vi "GT Get Dac Config.vi"(8 "error in (no error)":errorcluster caption="错误输入（无错误）", 9 "pDac":T1, 10 "dac":i16, 11 "cardNum":i16) -> (0 "error out":errorcluster caption="错误输出", 1 "pDac out":T1, 3 "function return":i16)   [LabVIEW 2020, in "gts1.lvlib"]
doc: "GT_API GT_GetDacConfig(short cardNum,short dac,TDacConfig *pDac);"
uses:
  gts1.lvlib
  dll/32bit/multi_card/gts.dll
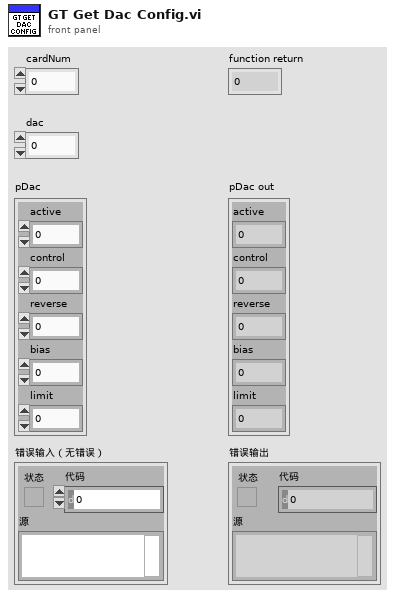
[diagram p1: front panel]
types:
  T1 = cluster{"active":i16, "control":i16, "reverse":i16, "bias":i16, "limit":i16}
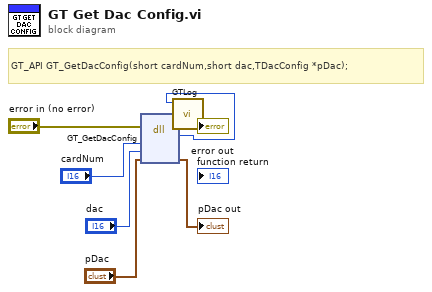
[diagram p0: block diagram]
diagram:
  # "GT_API GT_GetDacConfig(short cardNum,short dac,TDacConfig *pDac);"
  n1 = dll-call lib="C:/1228/dll/32bit/multi_card/gts.dll" fn="GT_GetDacConfig"(error in="error in (no error)", "cardNum"="cardNum", "dac"="dac", "pDac"="pDac") -> (error out=w3:errorcluster, w1:i16, "pDac"=→"pDac out":T1)  [unwired: 4 in, 1 out]
  n2 = call "GTLog.vi"("error in (no error)"=w3, "Numeric"=w1) -> ("error out"=→"error out":errorcluster)  [unwired: 9 in]
